vi "load_coating_(in).vi"() -> (1 "Recipe":string[](array[string]), 2 "Path Array":string[](array[string]))   [LabVIEW 2009]
uses:
  <vilib>/Utility/file.llb/Read From Spreadsheet File (string).vi
panel:
  out "string":string
  in  "Ok":bool caption="OK2"
  in  "Cancel":bool
  in  "Recipe List":i32(listbox)
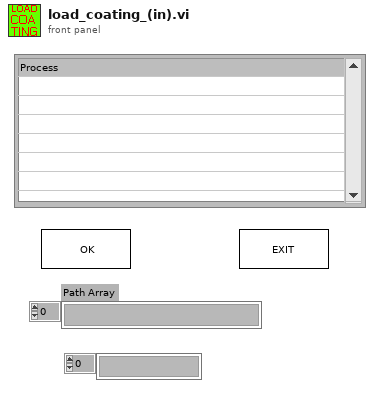
[diagram p1: front panel]
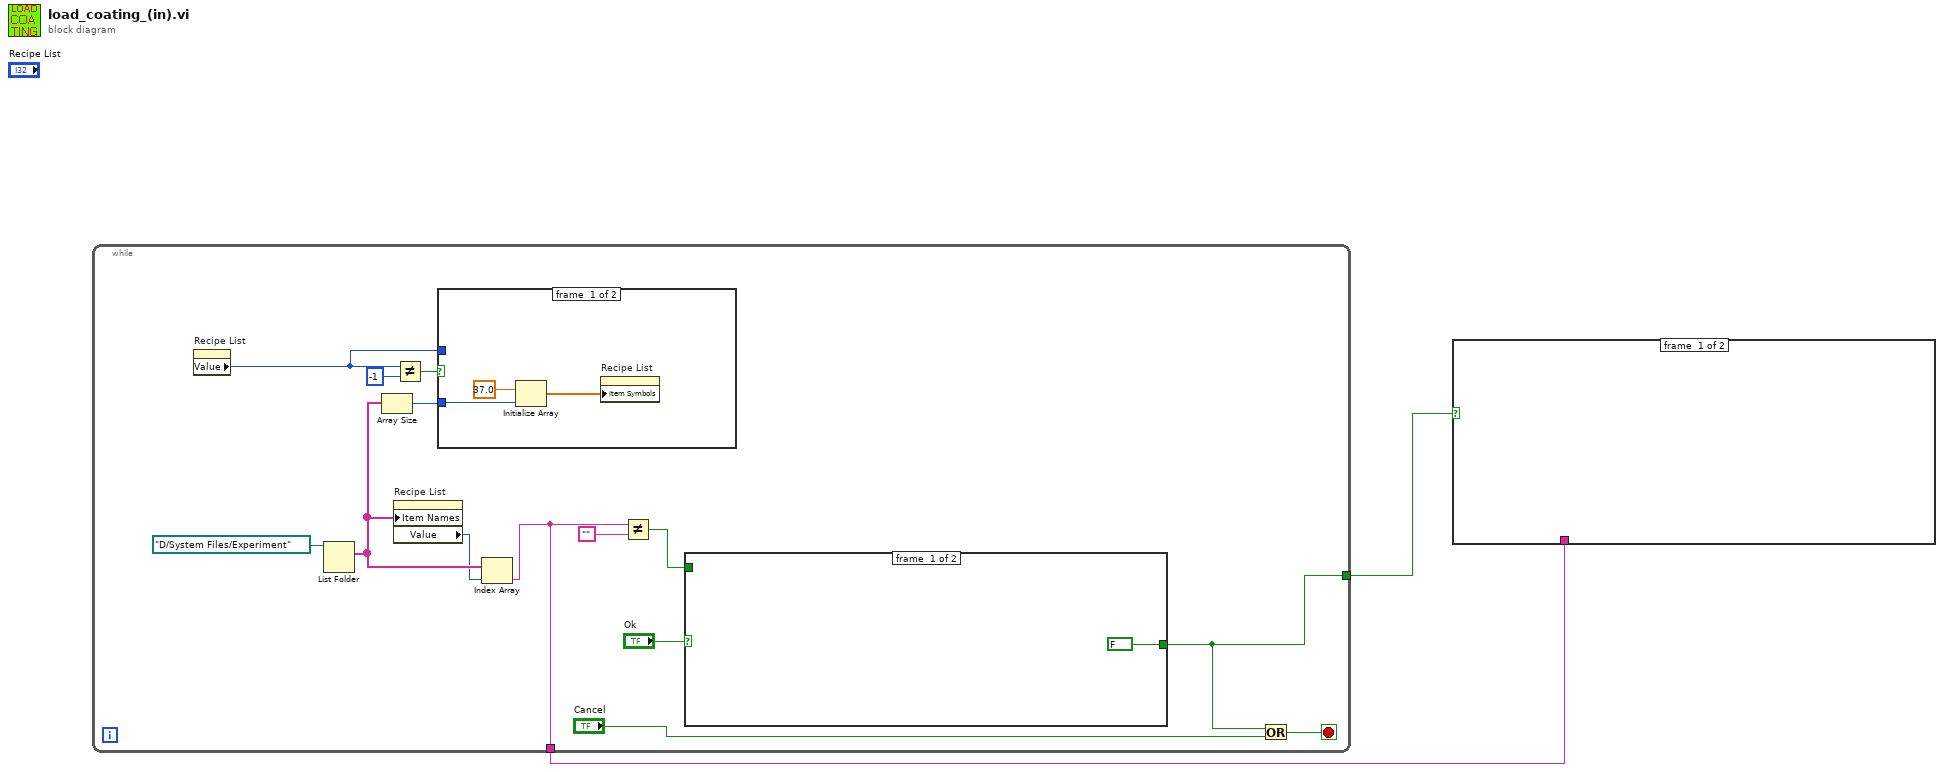
[diagram p0: block diagram]
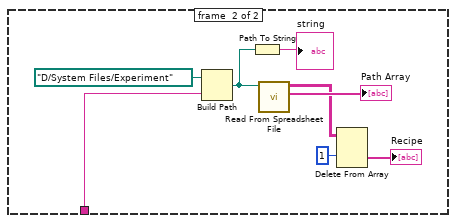
[diagram p2: hidden frame]
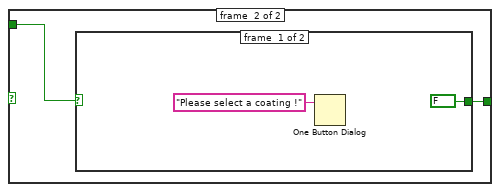
[diagram p3: hidden frame]
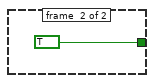
[diagram p4: hidden frame]
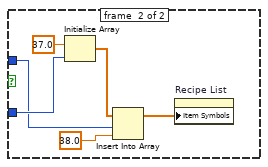
[diagram p5: hidden frame]
diagram:
  n1 = while {
    tunnel: [w3] -> w2
    tunnel: [w6] -> w1
    stop <- w7 stop-if-true
    n2 = property on="Recipe List" class="LstBox (strict)"() -> ("Value"=w12:i32)  [unwired: 2 in, 2 out]
    n3 = List Folder(path=path "D:/System Files/Experiment") -> (filenames=w11:string[])  [unwired: 3 in, 3 out]
    n4 = Array Size(array=w11) -> (size(s)=w13:i32)
    n5 = property on="Recipe List" class="LstBox (strict)"("Item Names"=w11) -> ("Value"=w10:i32)  [unwired: 2 in, 2 out]
    n6 = Not Equal?(x=w12, y=-1) -> (x != y?=w14:bool)
    n7 = case shown="True" w14 {
      tunnel: w13 -> [w24 w29]
      tunnel: w12 -> [_ w28]
      frame #0 {
        n8 = Initialize Array(37.0 ("element"), w24) -> (w23:dbl[])
        n9 = property on="Recipe List" class="LstBox (strict)"("Item Symbols"=w23) -> ()  [unwired: 2 in, 2 out]
      }
      frame #1 {
        n10 = Initialize Array(37.0 ("element"), w29) -> (w31:dbl[])
        n11 = Insert Into Array(array=w31, index=w28, new element=38.0 ("element")) -> (w26:dbl[])
        n12 = property on="Recipe List" class="LstBox (strict)"("Item Symbols"=w26) -> ()  [unwired: 2 in, 2 out]
      }
    }
    n13 = Index Array(array=w11, index=w10) -> (element=w6:string)
    n14 = Not Equal?(x=w6, y="") -> (x != y?=w4:bool)
    n15 = case shown="True" "Ok" {
      tunnel: w4 -> [_ w19]
      tunnel: [FALSE w18] -> w3
      frame #0 {
      }
      frame #1 {
        n16 = case shown="False" w19 {
          tunnel: [FALSE TRUE] -> w18
          frame #0 {
            n17 = One Button Dialog(message="Please select a coating !") -> ()  [unwired: 1 in, 1 out]
          }
          frame #1 {
          }
        }
      }
    }
    n18 = Or(x=w3, y="Cancel") -> (x .or. y?=w7:bool)
  }
  n19 = case shown="True" w2 {
    tunnel: w1 -> [_ w39]
    frame #0 {
    }
    frame #1 {
      n20 = Build Path(base path=path "D:/System Files/Experiment", name or relative path=w39) -> (appended path=w33:path)
      n21 = Path To String(path=w33) -> (string=→"string":string)
      n22 = call-poly <vilib>:"Read From Spreadsheet File.vi"("file path (dialog if empty)"=w33) -> ("first row"=→"Path Array":string[], "all rows"=w35:string[][])  [unwired: 6 in, 3 out]
      n23 = Delete From Array(array=w35, index (row)=1) -> (deleted portion=→"Recipe":string[])  [unwired: 2 in, 1 out]
    }
  }
